vi "Camera  IMAQdx Tester.vi"() -> ()   [LabVIEW 2017]
uses:
  Camera_IMAQdx_class/typedefs/Configuration--Cluster.ctl
  Camera_IMAQdx_class/Camera_IMAQdx.lvclass
  <userlib>/_OpenG.lib/comparison/comparison.llb/Boolean Changed__ogtk.vi
panel:
  in  "Refresh List":bool
  in  "Snap":bool
  in  "Start Stop Grab":bool
  in  "Connect to Camera":bool
  in  "Cameras":u16(ring) items=["VMware Virtual USB Video Device "]
  out "Image":T1(plugin-control)
  in  "OK":bool
  out "Frame Number:":u32
  out "Connected":bool
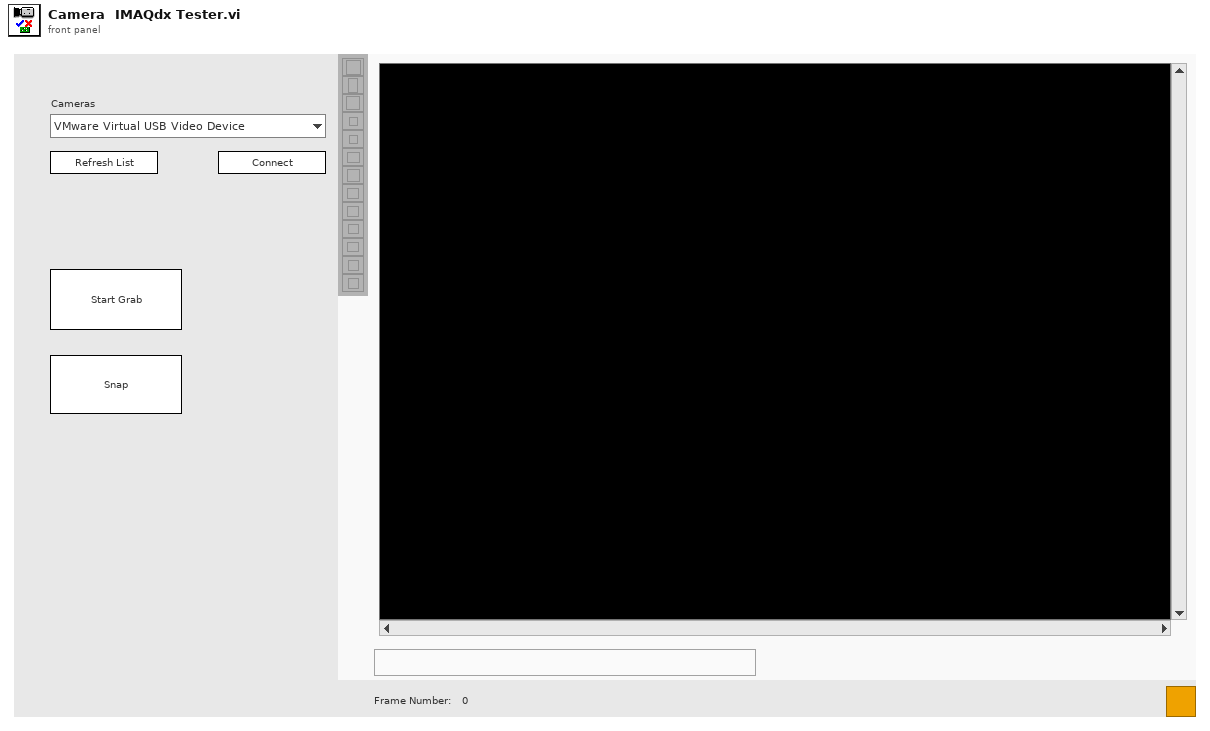
[diagram p1: front panel]
types:
  T1 = typedef "IMAQ Image.ctl" = refnum<image>
  T2 = typedef "Camera_IMAQdx.lvclass/Configuration--Cluster.ctl" = cluster{"Camera Interface Name":string, "Number of Buffers":u32, "Image Name":string, "Image Type":T3}
  T3 = typedef "Image Type" = u32
  T4 = enum32{"invalid app kind", "Development System", "Run Time System", "Student Edition", "Embedded LabVIEW", "Evaluation", "Custom"}
  T5 = enum8{"Enabled", "Disabled", "Disabled and Grayed Out"}
  T6 = enum32{"Invalid", "Standard", "Closed", "Hidden", "Minimized", "Maximized"}
  T7 = cluster{"Core":cluster{"Current VI Reference":refnum<vi>, "Close Panel on Exit?":bool}, "Camera.IMAQdx":refnum<class "Camera_IMAQdx.lvclass">, "All Camera Interfaces":string[], "Connected":bool, "Grabbing":bool}
  T8 = cluster{"Current VI Reference":refnum<vi>, "Close Panel on Exit?":bool}
  T9 = cluster{"Type":u32, "Version":u32, "Flags":u32, "SerialNumberHigh":u32, "SerialNumberLow":u32, "BusType":u32, "InterfaceName":string, "VendorName":string, "ModelName":string, "CameraFileName":string, "CameraAttributeURL":string}[]
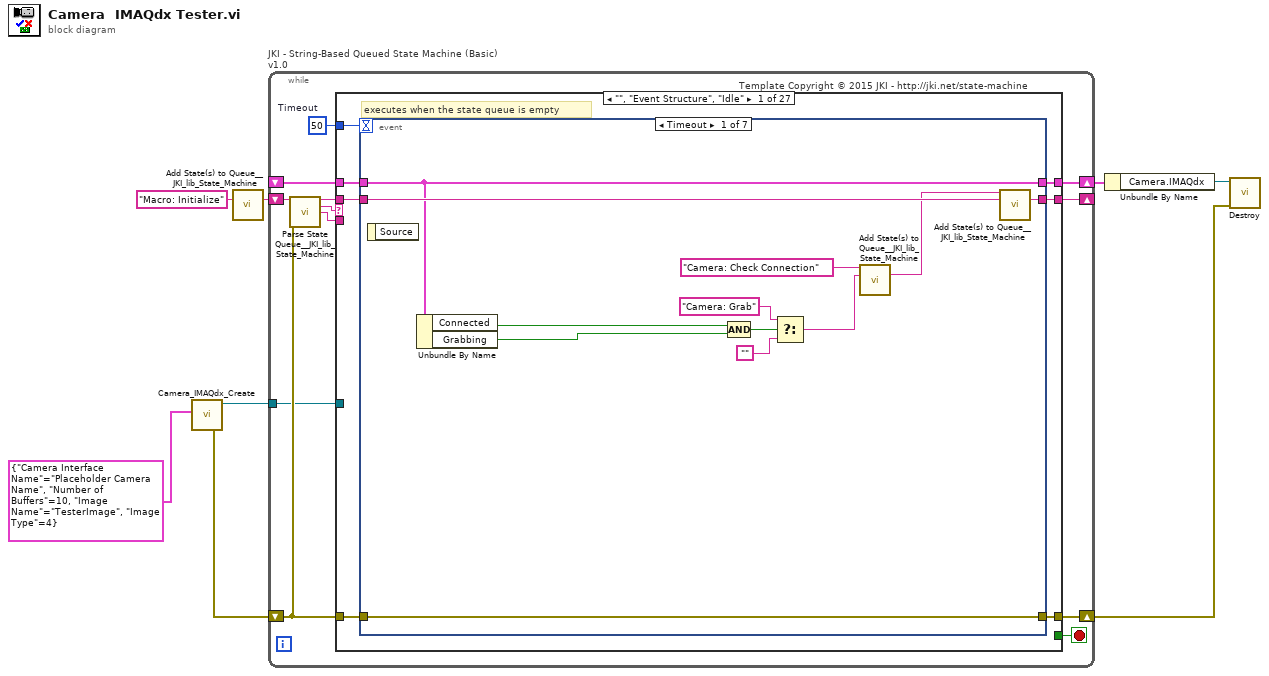
[diagram p0: block diagram]
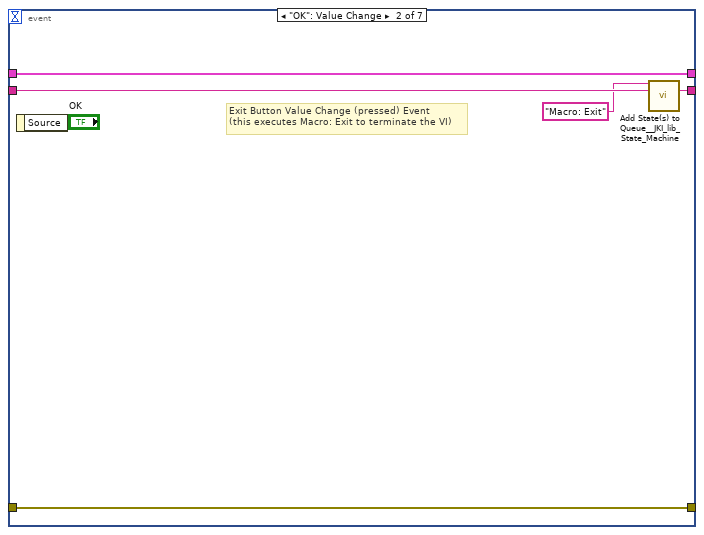
[diagram p2: hidden frame]
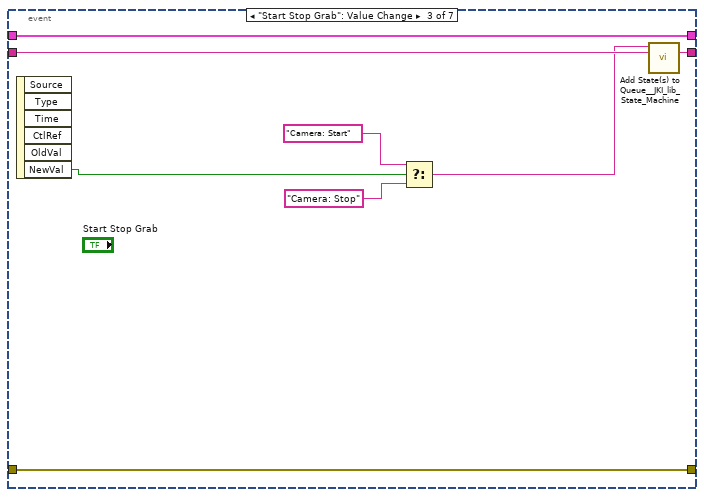
[diagram p3: hidden frame]
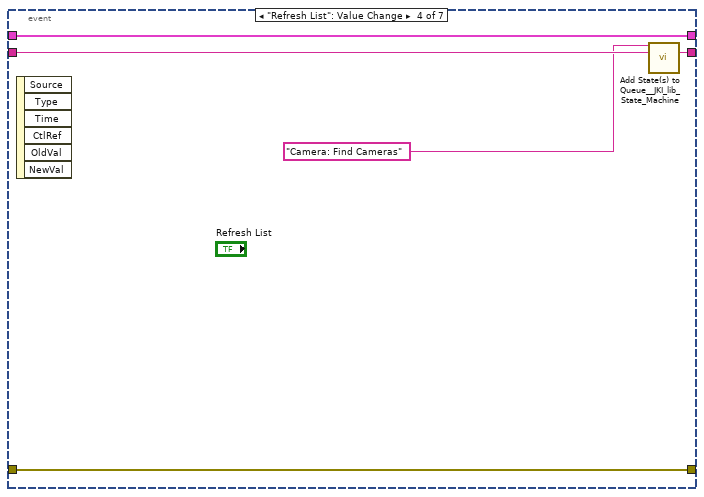
[diagram p4: hidden frame]
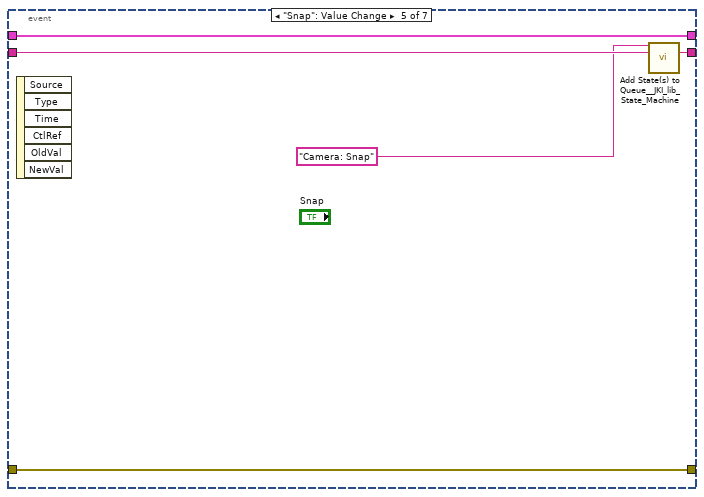
[diagram p5: hidden frame]
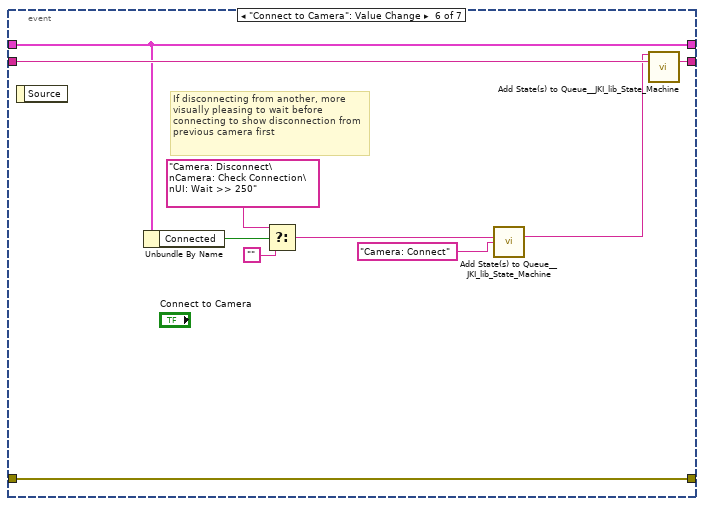
[diagram p6: hidden frame]
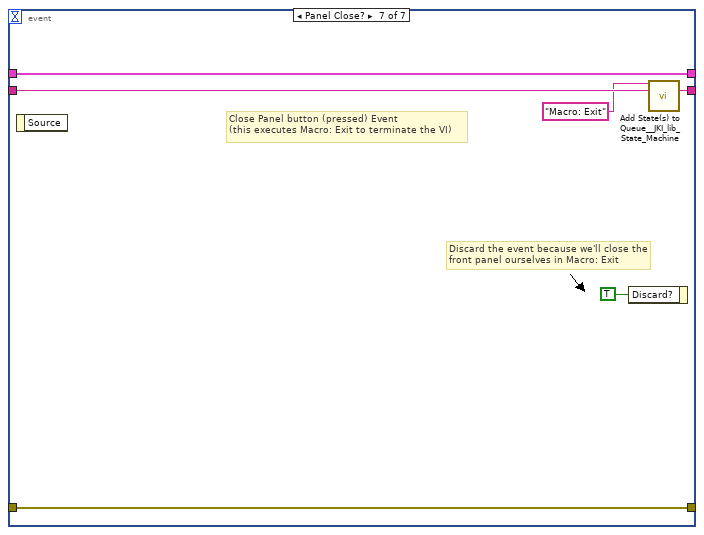
[diagram p7: hidden frame]
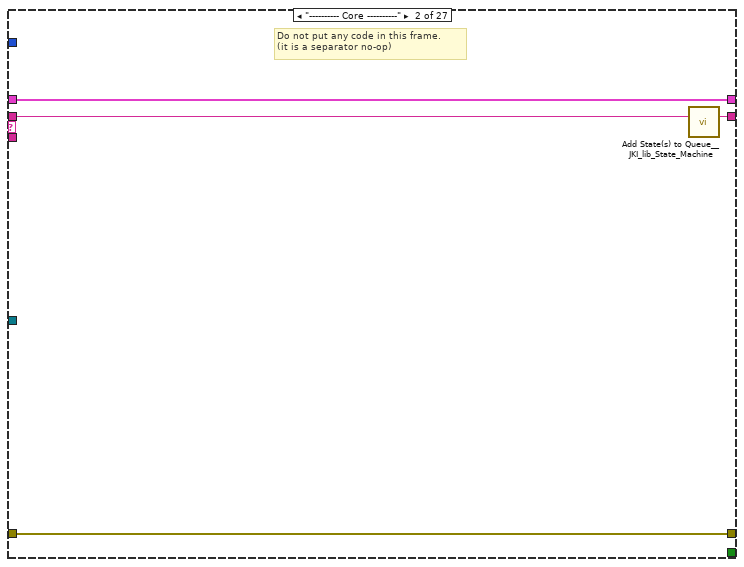
[diagram p8: hidden frame]
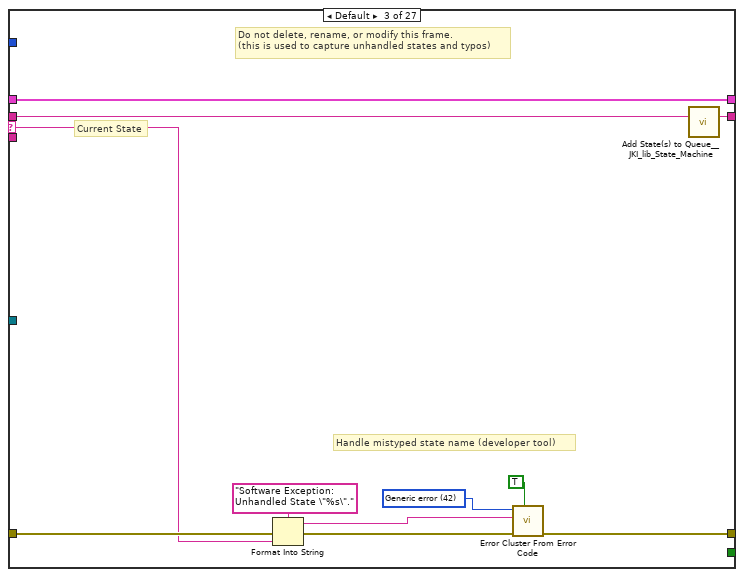
[diagram p9: hidden frame]
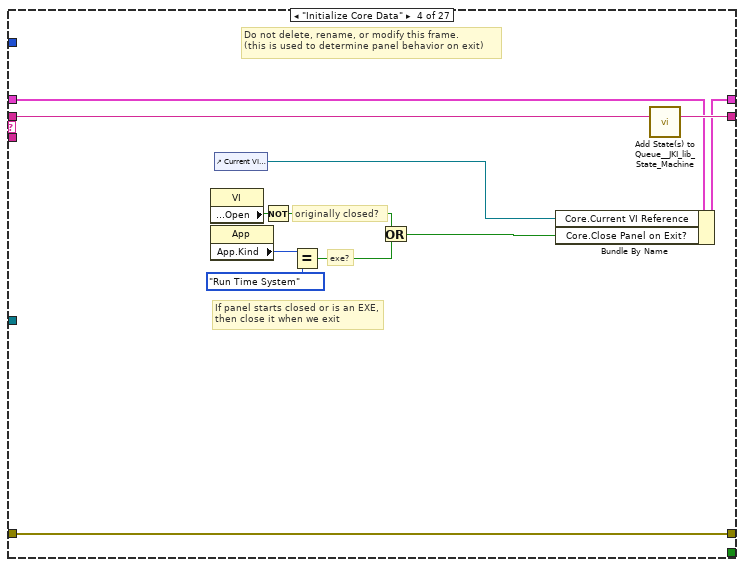
[diagram p10: hidden frame]
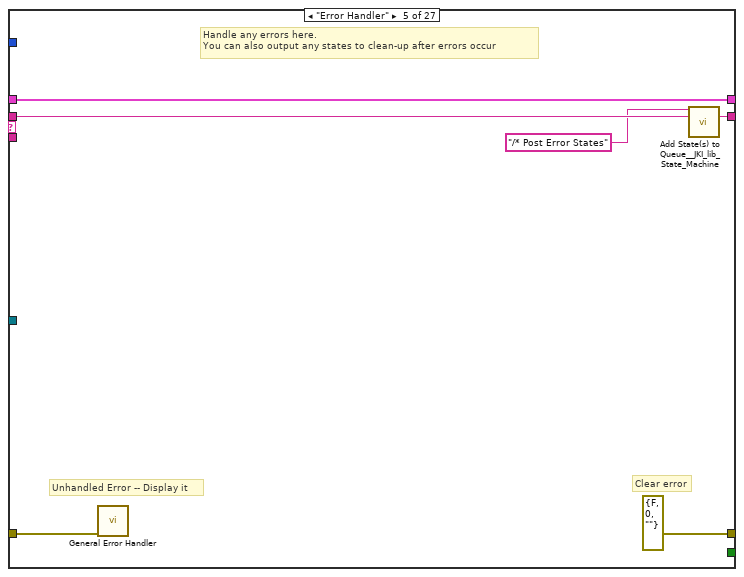
[diagram p11: hidden frame]
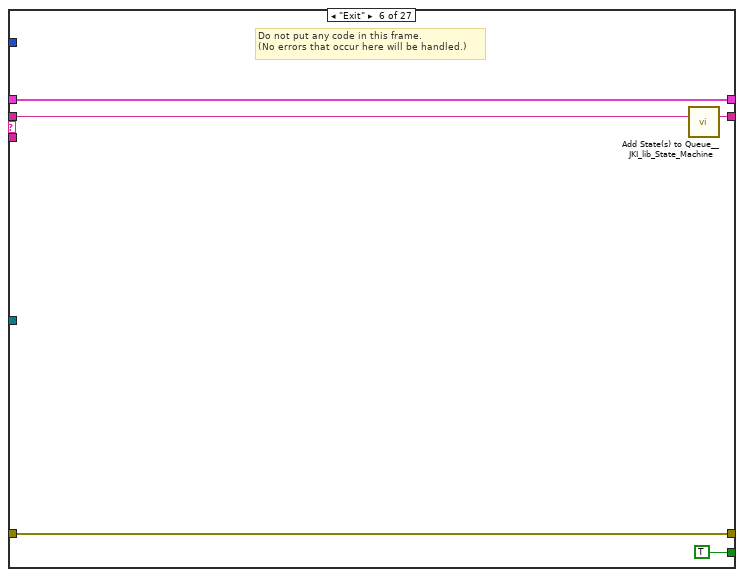
[diagram p12: hidden frame]
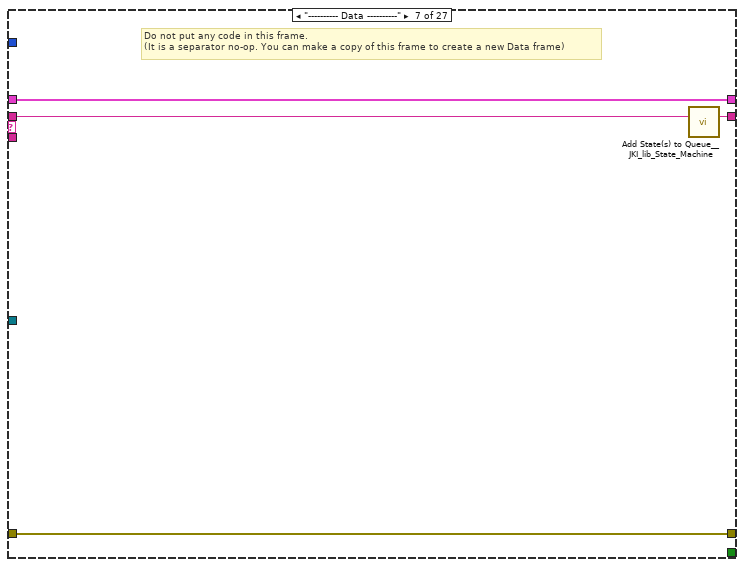
[diagram p13: hidden frame]
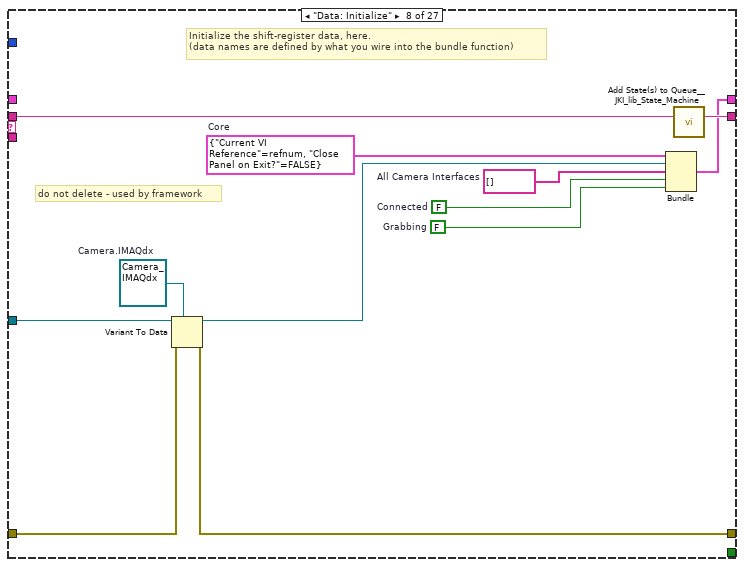
[diagram p14: hidden frame]
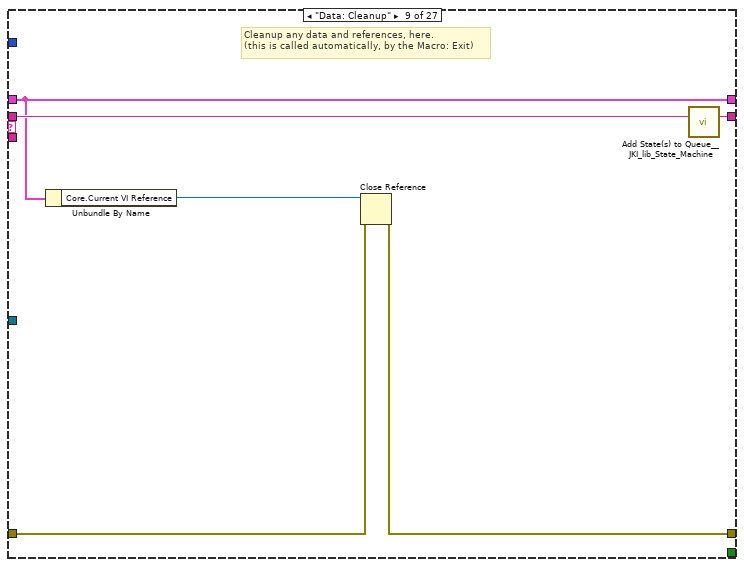
[diagram p15: hidden frame]
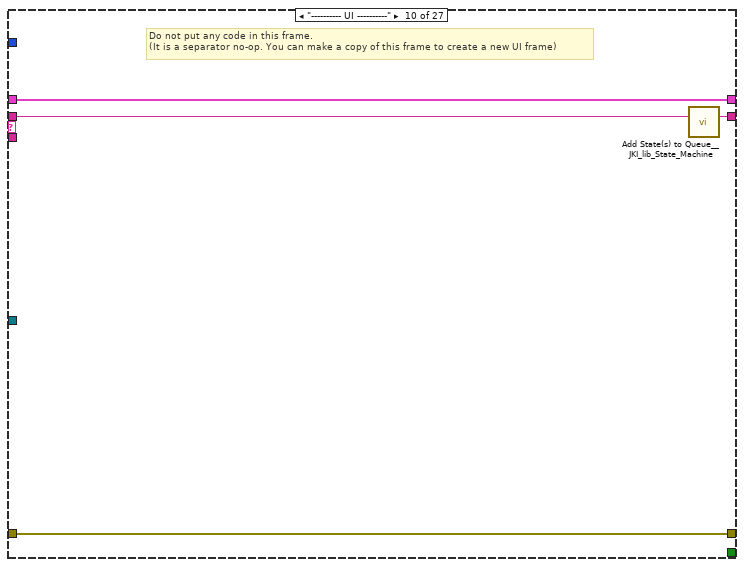
[diagram p16: hidden frame]
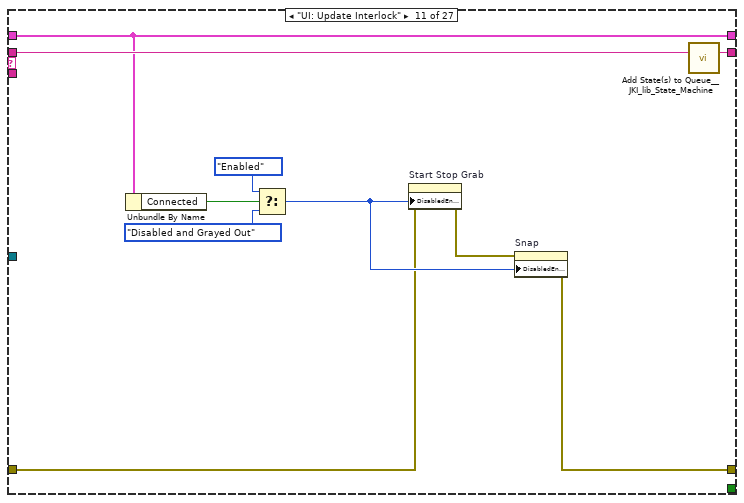
[diagram p17: hidden frame]
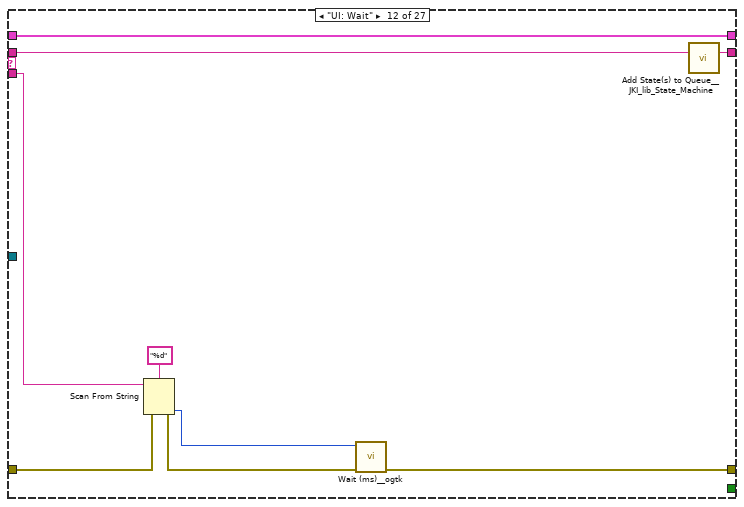
[diagram p18: hidden frame]
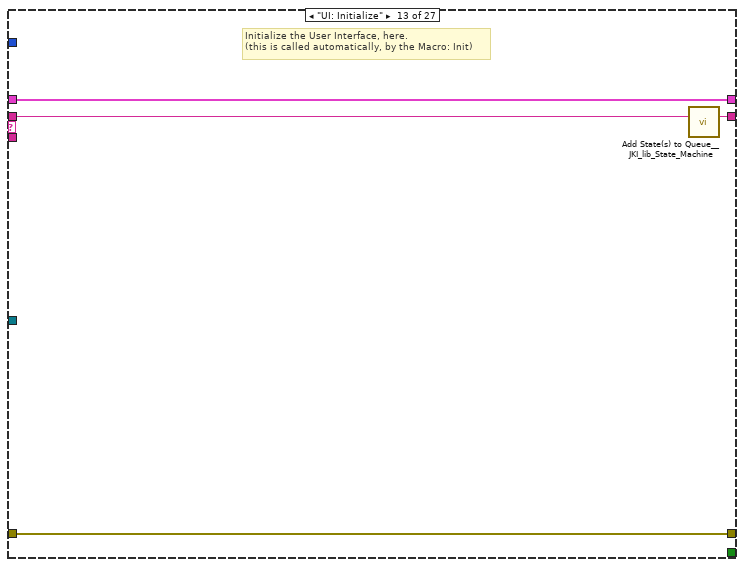
[diagram p19: hidden frame]
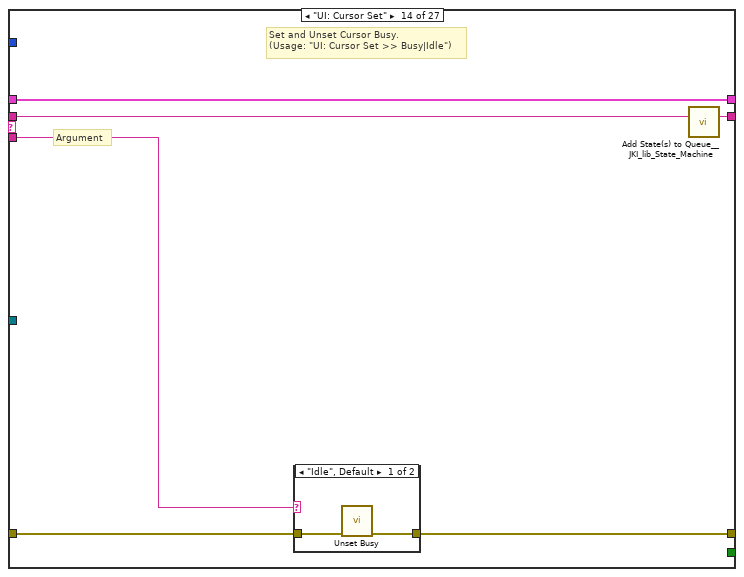
[diagram p20: hidden frame]
diagram:
  n1 = call "Camera_IMAQdx_Create.vi"("Configuration"=T2 {"Camera Interface Name"="Placeholder Camera Name", "Number of Buffers"=10, "Image Name"="TesterImage", "Image Type"=4}) -> ("error out"=w3:errorcluster, "reference out"=w6:refnum<class "Camera_IMAQdx.lvclass">)  [unwired: 9 in]
  n2 = call <vilib>:"Add State(s) to Queue__JKI_lib_State_Machine.vi"("State(s) in (\"\")"="Macro: Initialize") -> ("States Out"=w8:string)  [unwired: 14 in]
  n3 = while "JKI - String-Based Queued State Machine (Basic) v1.0" {
    shift-right: [w13] -> w5
    shift-left: _ -> [w12]
    shift-right: [w16] -> w2
    shift-left: w3 -> [w10]
    shift-right: [w15] -> _
    shift-left: w8 -> [w17]
    tunnel: w6 -> [w9]
    stop <- w14 stop-if-true
    w11 = 50  # Timeout
    # "Template Copyright © 2015 JKI - http://jki.net/state-machine"
    n4 = call <vilib>:"Parse State Queue__JKI_lib_State_Machine.vi"("State Queue"=w17, "Error In (no error)"=w10) -> ("Remaining States"=w19:string, "Current State"=w20:string, "Arguments"=w18:string)  [unwired: 11 in]
    n5 = case shown="\"\", \"Event Structure\", \"Idle\"" w20 {
      selector: w20 -> [_ _ w83 _ _ _ _ _ _ _ _ _ _ _ _ _ _ _ _ _ _ _ _ _ _ _ _]
      tunnel: w19 -> [w27 w82 w87 w105 w111 w116 w120 w132 w138 w142 w152 w161 w165 w171 w182 w208 w213 w232 w236 w244 w251 w263 w272 w281 w292 w309 w315]
      tunnel: w18 -> [_ _ _ _ _ _ _ _ _ _ _ w157 _ w166 w176 _ _ _ _ _ _ _ _ _ _ _ _]
      tunnel: w12 -> [w25 w79 w85 w96 w108 w114 w117 _ w133 w139 w150 w159 w163 w169 w178 w205 w210 w229 w233 w242 w249 w258 w265 w276 w284 w307 w313]
      tunnel: [w24 w80 w89 w102 errorcluster {"status"=FALSE, "code"=0, "source"=""} ("error out") w113 w118 w123 w134 w140 w143 w158 w162 w167 w179 w206 w211 w230 w234 w239 w246 w259 w268 w277 w287 w299 w310] -> w16
      tunnel: w10 -> [w23 w80 w88 w102 w107 w113 w118 w124 w135 w140 w144 w154 w162 w168 w180 w206 w211 w230 w234 w240 w247 w260 w269 w278 w286 w301 w311]
      tunnel: [w26 w81 w86 w104 w110 w115 w119 w131 w137 w141 w151 w160 w164 w170 w181 w207 w212 w231 w235 w243 w250 w262 w271 w280 w291 w308 w314] -> w15
      tunnel: [_ _ _ _ _ TRUE _ _ _ _ _ _ _ _ _ _ _ _ _ _ _ _ _ _ _ _ _] -> w14
      tunnel: [w22 w79 w85 w103 w108 w114 w117 w130 w133 w139 w150 w159 w163 w169 w178 w205 w210 w229 w233 w242 w249 w257 w264 w275 w283 w307 w313] -> w13
      tunnel: w11 -> [w21 _ _ _ _ _ _ _ _ _ _ _ _ _ _ _ _ _ _ _ _ _ _ _ _ _ _]
      tunnel: w9 -> [_ _ _ _ _ _ _ w128 _ _ _ _ _ _ _ _ _ _ _ _ _ _ _ _ _ _ _]
      frame "", "Event Structure", "Idle" {
        # "executes when the state queue is empty"
        n6 = event shown="[0] Timeout" {
          selector: _ -> [_ _ _ _ _ _ _]
          dyn-events: _ -> [_ _ _ _ _ _ _]
          timeout: w21 -> [_ _ _ _ _ _ _]
          tunnel: w27 -> [w39 w44 w52 w57 w62 w72 w78]
          tunnel: [w38 w43 w51 w56 w61 w71 w77] -> w26
          tunnel: w25 -> [w36 w41 w49 w54 w59 w69 w75]
          tunnel: [w37 w42 w50 w55 w60 w70 w76] -> w24
          tunnel: w23 -> [w37 w42 w50 w55 w60 w70 w76]
          tunnel: [w36 w41 w49 w54 w59 w69 w75] -> w22
          event Timeout {
            n7 = event-data() -> ()  [unwired: 1 in, 1 out]
            n8 = Unbundle By Name(w36) -> ("Connected"=w35:bool, "Grabbing"=w34:bool)
            n9 = Compound Arithmetic op=AND(w35, w34) -> (w33:bool)
            n10 = Select(t="Camera: Grab", s=w33, f="") -> (s? t:f=w28:string)
            n11 = call <vilib>:"Add State(s) to Queue__JKI_lib_State_Machine.vi"("State(s) in Front (\"\")"="Camera: Check Connection", "State(s) in (\"\")"=w28) -> ("States Out"=w29:string)  [unwired: 13 in]
            n12 = call <vilib>:"Add State(s) to Queue__JKI_lib_State_Machine.vi"("State(s) in Front (\"\")"=w29, "State(s) in (\"\")"=w39) -> ("States Out"=w38:string)  [unwired: 13 in]
          }
          event "OK": Value Change {
            # "Exit Button Value Change (pressed) Event\n(this executes Macro: Exit to terminate the VI)"
            n13 = event-data() -> ()  [unwired: 1 in, 1 out]
            n14 = call <vilib>:"Add State(s) to Queue__JKI_lib_State_Machine.vi"("State(s) in Front (\"\")"="Macro: Exit", "State(s) in (\"\")"=w44) -> ("States Out"=w43:string)  [unwired: 13 in]
          }
          event "Start Stop Grab": Value Change {
            n15 = event-data() -> ("NewVal"=w46:bool)  [unwired: 1 in, 5 out]
            n16 = Select(t="Camera: Start", s=w46, f="Camera: Stop") -> (s? t:f=w45:string)
            n17 = call <vilib>:"Add State(s) to Queue__JKI_lib_State_Machine.vi"("State(s) in Front (\"\")"=w45, "State(s) in (\"\")"=w52) -> ("States Out"=w51:string)  [unwired: 13 in]
          }
          event "Refresh List": Value Change {
            n18 = event-data() -> ()  [unwired: 1 in, 6 out]
            n19 = call <vilib>:"Add State(s) to Queue__JKI_lib_State_Machine.vi"("State(s) in Front (\"\")"="Camera: Find Cameras", "State(s) in (\"\")"=w57) -> ("States Out"=w56:string)  [unwired: 13 in]
          }
          event "Snap": Value Change {
            n20 = event-data() -> ()  [unwired: 1 in, 6 out]
            n21 = call <vilib>:"Add State(s) to Queue__JKI_lib_State_Machine.vi"("State(s) in Front (\"\")"="Camera: Snap", "State(s) in (\"\")"=w62) -> ("States Out"=w61:string)  [unwired: 13 in]
          }
          event "Connect to Camera": Value Change {
            # "If disconnecting from another, more visually pleasing to wait before connecting to show disconnection from previous camera first"
            n22 = event-data() -> ()  [unwired: 1 in, 1 out]
            n23 = Unbundle By Name(w69) -> ("Connected"=w68:bool)
            n24 = Select(t="Camera: Disconnect\nCamera: Check Connection\nUI: Wait >> 250", s=w68, f="") -> (s? t:f=w65:string)
            n25 = call <vilib>:"Add State(s) to Queue__JKI_lib_State_Machine.vi"("State(s) in (\"\")"=w65, "State(s) at Back (\"\")"="Camera: Connect") -> ("States Out"=w63:string)  [unwired: 13 in]
            n26 = call <vilib>:"Add State(s) to Queue__JKI_lib_State_Machine.vi"("State(s) in Front (\"\")"=w63, "State(s) in (\"\")"=w72) -> ("States Out"=w71:string)  [unwired: 13 in]
          }
          event Panel Close? {
            # "Discard the event because we'll close the front panel ourselves in Macro: Exit"
            # "Close Panel button (pressed) Event\n(this executes Macro: Exit to terminate the VI)"
            n27 = event-data() -> ()  [unwired: 1 in, 1 out]
            n28 = event-data("Discard?"=TRUE) -> ()  [unwired: 1 in, 1 out]
            n29 = call <vilib>:"Add State(s) to Queue__JKI_lib_State_Machine.vi"("State(s) in Front (\"\")"="Macro: Exit", "State(s) in (\"\")"=w78) -> ("States Out"=w77:string)  [unwired: 13 in]
          }
        }
      }
      frame "---------- Core ----------" {
        # "Do not put any code in this frame.\n(it is a separator no-op)"
        n30 = call <vilib>:"Add State(s) to Queue__JKI_lib_State_Machine.vi"("State(s) in (\"\")"=w82) -> ("States Out"=w81:string)  [unwired: 14 in]
      }
      frame Default {
        w92 = 42 items=["No error", "Argument error", "Memory is full", "Out of zone", "End of file", "File already open", "Generic file I/O error", "File not found", "File permission error", "Disk is full", "Duplicate path", "Too many files open", "System feature not enabled", "Resource file not found", "Cannot add resource", "Resource not found", "Image not found", "Image memory error", "Pen does not exist", "Config type invalid", "Config token not found", "Config parse error", "Config memory error", "Bad external code format", "Bad external code offset", "External code not present", "Null window", "Destroy window error", "Null menu", "Print aborted", "Bad print record", "Print driver error", "Windows error during printing", "Memory error during printing", "Print dialog error", "Generic print error", "Invalid device refnum", "Device not found", "Device parameter error", "Device unit error", "Cannot open device", "Device call aborted", "Generic error", "Cancelled by user", "Object ID too low", "Object ID too high", "Object not in heap", "Unknown heap", "Unknown object (invalid DefProc)", "Unknown object (DefProc not in table)", "Message out of range", "Invalid (null) method", "Unknown message", "Manager call not supported", "Bad address", "Network operation in progress", "Network operation timed out", "Connection is busy", "Network attribute not supported", "Network error", "Address in use", "System out of memory", "Connection aborted", "Connection refused", "Not connected", "Already connected", "Connection closed", "Initialization error (interapplication manager)", "Bad occurrence", "Wait on unbound occurrence handler", "Occurrence queue overflow", "Datalog type conflict", "Unused", "Unrecognized type (interapplication manager)", "Memory corrupt", "Failed to make temporary DLL", "Old CIN version", "Drag socket not found", "Failed to load drop-object", "Failed to register OLE object", "Failed to release OLE object", "Format specifier type mismatch", "Unknown format specifier", "Too few format specifiers", "Too many format specifiers", "Scan failed", "Newer CIN version", "Error converting to variant", "Runtime menu error", "Password tampered", "Variant attribute not found", "Incompatible variant data type", "Event data is not available", "Event Store is not present", "Occurrence is not found", "Event Queue is not created", "Event info is not available", "Refnum passed is NULL", "Error retrieving Class GUID", "Error retrieving CoClass GUID", "Error retrieving TypeLib GUID.", "Bad built application magic bytes.", "Specific driver is different from the specific driver associated with the Logical Name.", "There is no session opened to the class driver.", "Max Error", "MAX - Error with config objects", "MAX - Error loading configuration", "MAX - Group not supported"]
        # "Current State"
        # "Do not delete, rename, or modify this frame.\n(this is used to capture unhandled states and typos)"
        # "Handle mistyped state name (developer tool)"
        n31 = Format Into String(format string="Software Exception: Unhandled State \"%s\"." ("message"), error in=w88, w83) -> (resulting string=w91:string, error out=w90:errorcluster)  [unwired: 1 in]
        n32 = call <vilib>:"Error Cluster From Error Code.vi"("show call chain? (False)"=TRUE, "error in (no error)"=w90, "error message (\"\")"=w91, "error code (0)"=w92) -> ("error out"=w89:errorcluster)  [unwired: 5 in]
        n33 = call <vilib>:"Add State(s) to Queue__JKI_lib_State_Machine.vi"("State(s) in (\"\")"=w87) -> ("States Out"=w86:string)  [unwired: 14 in]
      }
      frame "Initialize Core Data" {
        # "Do not delete, rename, or modify this frame.\n(this is used to determine panel behavior on exit)"
        # "originally closed?"
        # "exe?"
        # "If panel starts closed or is an EXE, then close it when we exit"
        n34 = property class="VI"() -> ("Front Panel.Open"=w101:bool)  [unwired: 2 in, 2 out]
        n35 = property class="App"() -> ("App.Kind"=w100:T4)  [unwired: 2 in, 2 out]
        n36 = control-ref of="Current VI Reference"() -> (w94:refnum<vi>)
        n37 = Not(x=w101) -> (.not. x?=w98:bool)
        n38 = Equal?(x=w100, y=T4."Run Time System" ("Application:Kind")) -> (x = y?=w97:bool)
        n39 = Or(x=w98, y=w97) -> (x .or. y?=w95:bool)
        n40 = Bundle By Name(cluster=w96, "Core.Current VI Reference"=w94, "Core.Close Panel on Exit?"=w95) -> (w103:T7)
        n41 = call <vilib>:"Add State(s) to Queue__JKI_lib_State_Machine.vi"("State(s) in (\"\")"=w105) -> ("States Out"=w104:string)  [unwired: 14 in]
      }
      frame "Error Handler" {
        # "Unhandled Error -- Display it"
        # "Handle any errors here.\nYou can also output any states to clean-up after errors occur"
        # "Clear error"
        n42 = call <vilib>:"General Error Handler.vi"("error in (no error)"=w107) -> ()  [unwired: 10 in, 5 out]
        n43 = call <vilib>:"Add State(s) to Queue__JKI_lib_State_Machine.vi"("State(s) in Front (\"\")"="/* Post Error States", "State(s) in (\"\")"=w111) -> ("States Out"=w110:string)  [unwired: 13 in]
      }
      frame "Exit" {
        # "Do not put any code in this frame.\n(No errors that occur here will be handled.)"
        n44 = call <vilib>:"Add State(s) to Queue__JKI_lib_State_Machine.vi"("State(s) in (\"\")"=w116) -> ("States Out"=w115:string)  [unwired: 14 in]
      }
      frame "---------- Data ----------" {
        # "Do not put any code in this frame.\n(It is a separator no-op. You can make a copy of this frame to create a new Data frame)"
        n45 = call <vilib>:"Add State(s) to Queue__JKI_lib_State_Machine.vi"("State(s) in (\"\")"=w120) -> ("States Out"=w119:string)  [unwired: 14 in]
      }
      frame "Data: Initialize" {
        w121 = FALSE  # Grabbing
        w122 = FALSE  # Connected
        w126 = refnum<class "Camera_IMAQdx.lvclass"> refnum  # Camera.IMAQdx
        w127 = string[] []  # All Camera Interfaces
        w129 = T8 {"Current VI Reference"=refnum, "Close Panel on Exit?"=FALSE}  # Core
        # "do not delete - used by framework"
        # "Initialize the shift-register data, here.\n(data names are defined by what you wire into the bundle function)"
        n46 = Variant To Data(error in=w124, type=w126, Variant=w128) -> (data=w125:refnum<class "Camera_IMAQdx.lvclass">, error out=w123:errorcluster)
        n47 = Bundle("Core"=w129, "Camera.IMAQdx"=w125, "All Camera Interfaces"=w127, "Connected"=w122, "Grabbing"=w121) -> (w130:T7)  [unwired: 1 in]
        n48 = call <vilib>:"Add State(s) to Queue__JKI_lib_State_Machine.vi"("State(s) in (\"\")"=w132) -> ("States Out"=w131:string)  [unwired: 14 in]
      }
      frame "Data: Cleanup" {
        # "Cleanup any data and references, here.\n(this is called automatically, by the Macro: Exit)"
        n49 = Unbundle By Name(w133) -> ("Core.Current VI Reference"=w136:refnum<vi>)
        n50 = Close Reference(reference=w136, error in (no error)=w135) -> (error out=w134:errorcluster)
        n51 = call <vilib>:"Add State(s) to Queue__JKI_lib_State_Machine.vi"("State(s) in (\"\")"=w138) -> ("States Out"=w137:string)  [unwired: 14 in]
      }
      frame "---------- UI ----------" {
        # "Do not put any code in this frame.\n(It is a separator no-op. You can make a copy of this frame to create a new UI frame)"
        n52 = call <vilib>:"Add State(s) to Queue__JKI_lib_State_Machine.vi"("State(s) in (\"\")"=w142) -> ("States Out"=w141:string)  [unwired: 14 in]
      }
      frame "UI: Update Interlock" {
        n53 = Unbundle By Name(w150) -> ("Connected"=w149:bool)
        n54 = Select(t=T5."Enabled" ("Disabled"), s=w149, f=T5."Disabled and Grayed Out" ("Disabled")) -> (s? t:f=w146:T5)
        n55 = property on="Start Stop Grab" class="Bool (strict)"(error in=w144, "DisabledEnum"=w146) -> (error out=w145:errorcluster)  [unwired: 1 in, 1 out]
        n56 = property on="Snap" class="Bool"(error in=w145, "DisabledEnum"=w146) -> (error out=w143:errorcluster)  [unwired: 1 in, 1 out]
        n57 = call <vilib>:"Add State(s) to Queue__JKI_lib_State_Machine.vi"("State(s) in (\"\")"=w152) -> ("States Out"=w151:string)  [unwired: 14 in]
      }
      frame "UI: Wait" {
        n58 = Scan From String(format string="%d", input string=w157, error in=w154) -> (error out=w153:errorcluster, output 1=w155:i32)  [unwired: 2 in, 2 out]
        n59 = call <userlib>:"Wait (ms)__ogtk.vi"("error in (no error)"=w153, "milliseconds to wait"=w155) -> ("error out"=w158:errorcluster)  [unwired: 8 in, 1 out]
        n60 = call <vilib>:"Add State(s) to Queue__JKI_lib_State_Machine.vi"("State(s) in (\"\")"=w161) -> ("States Out"=w160:string)  [unwired: 14 in]
      }
      frame "UI: Initialize" {
        # "Initialize the User Interface, here.\n(this is called automatically, by the Macro: Init)"
        n61 = call <vilib>:"Add State(s) to Queue__JKI_lib_State_Machine.vi"("State(s) in (\"\")"=w165) -> ("States Out"=w164:string)  [unwired: 14 in]
      }
      frame "UI: Cursor Set" {
        # "Argument"
        # "Set and Unset Cursor Busy.\n(Usage: \"UI: Cursor Set >> Busy|Idle\")"
        n62 = case shown="\"Idle\", Default" w166 {
          tunnel: w168 -> [w173 w175]
          tunnel: [w172 w174] -> w167
          frame "Idle", Default {
            n63 = call <vilib>:"Unset Busy.vi"("error in (no error)"=w173) -> ("error out"=w172:errorcluster)  [unwired: 10 in]
          }
          frame "Busy" {
            n64 = call <vilib>:"Set Busy.vi"("error in (no error)"=w175) -> ("error out"=w174:errorcluster)  [unwired: 9 in, 1 out]
          }
        }
        n65 = call <vilib>:"Add State(s) to Queue__JKI_lib_State_Machine.vi"("State(s) in (\"\")"=w171) -> ("States Out"=w170:string)  [unwired: 14 in]
      }
      frame "UI: Front Panel State" {
        # "Argument"
        # "Set Front Panel Open or Closed\n(Usage: \"UI: Front Panel State >> Open|Close\")"
        n66 = Unbundle By Name(w178) -> ("Core.Current VI Reference"=w177:refnum<vi>)
        n67 = case shown="\"Open\", Default" w176 {
          tunnel: w180 -> [w186 w199]
          tunnel: [w188 w200] -> w179
          tunnel: w177 -> [w187 w197]
          frame "Open", Default {
            n68 = property class="VI"(reference=w187, error in=w186) -> (reference out=w184:refnum<vi>, error out=w185:errorcluster, "Front Panel.Open"=w183:bool)
            n69 = case shown="False" w183 {
              tunnel: [w191 w194] -> w188
              tunnel: w185 -> [w190 w194]
              tunnel: w184 -> [w189 _]
              frame False {
                n70 = invoke class="VI" method="FP.Open"(reference=w189, error in=w190, "Activate"=TRUE, "State"=T6."Standard") -> (error out=w191:errorcluster)  [unwired: 1 in, 4 out]
              }
              frame True {
              }
            }
          }
          frame "Close" {
            n71 = property class="VI"(reference=w197, error in=w199) -> (reference out=w196:refnum<vi>, error out=w198:errorcluster, "Front Panel.Open"=w195:bool)
            n72 = case shown="True" w195 {
              tunnel: [w201 w204] -> w200
              tunnel: w198 -> [w201 w203]
              tunnel: w196 -> [_ w202]
              frame False {
              }
              frame True {
                n73 = invoke class="VI" method="FP.Close"(reference=w202, error in=w203) -> (error out=w204:errorcluster)  [unwired: 1 in, 2 out]
              }
            }
          }
        }
        n74 = call <vilib>:"Add State(s) to Queue__JKI_lib_State_Machine.vi"("State(s) in (\"\")"=w182) -> ("States Out"=w181:string)  [unwired: 14 in]
      }
      frame "---------- Macro ----------" {
        # "Do not put any code in this frame.\n(It is a separator no-op. You can make a copy of this frame to create a new Macro frame)"
        n75 = call <vilib>:"Add State(s) to Queue__JKI_lib_State_Machine.vi"("State(s) in (\"\")"=w208) -> ("States Out"=w207:string)  [unwired: 14 in]
      }
      frame "Macro: Initialize" {
        # "Initialization Macro\n(This is called once, when the VI starts)"
        n76 = call <vilib>:"Add State(s) to Queue__JKI_lib_State_Machine.vi"("State(s) in Front (\"\")"="Data: Initialize\nInitialize Core Data\nUI: Initialize\nCamera: Find Cameras\nUI: Update Interlock\nUI: Front Panel State >> Open", "State(s) in (\"\")"=w213) -> ("States Out"=w212:string)  [unwired: 13 in]
      }
      frame "Macro: Exit" {
        # "Exit Macro\n(This is called once, when the VI exits)"
        n77 = Unbundle By Name(w229) -> ("Grabbing"=w218:bool, "Connected"=w217:bool, "Core.Close Panel on Exit?"=w228:bool)
        n78 = Select(t="Camera: Stop", s=w218, f="") -> (s? t:f=w216:string)
        n79 = Select(t="Camera: Disconnect", s=w217, f="") -> (s? t:f=w215:string)
        n80 = Select(t="UI: Front Panel State >> Close", s=w228, f="") -> (s? t:f=w225:string)
        n81 = call <vilib>:"Add State(s) to Queue__JKI_lib_State_Machine.vi"("State(s) in Front (\"\")"=w216, "State(s) in (\"\")"=w215) -> ("States Out"=w214:string)  [unwired: 13 in]
        n82 = call <vilib>:"Add State(s) to Queue__JKI_lib_State_Machine.vi"("State(s) in Front (\"\")"=w214, "State(s) in (\"\")"=w225, "State(s) at Back (\"\")"="Data: Cleanup\nExit") -> ("States Out"=w223:string)  [unwired: 12 in]
        n83 = call <vilib>:"Add State(s) to Queue__JKI_lib_State_Machine.vi"("State(s) in Front (\"\")"=w223, "State(s) in (\"\")"=w232) -> ("States Out"=w231:string)  [unwired: 13 in]
      }
      frame "---------- Camera ----------" {
        # "Template Separator\n(You can make a copy of, or modify, this frame)"
        n84 = call <vilib>:"Add State(s) to Queue__JKI_lib_State_Machine.vi"("State(s) in (\"\")"=w236) -> ("States Out"=w235:string)  [unwired: 14 in]
      }
      frame "Camera: Grab" {
        n85 = Unbundle By Name(w242) -> ("Camera.IMAQdx"=w241:refnum<class "Camera_IMAQdx.lvclass">)
        n86 = call-dynamic "Grab.vi"("error in (no error)"=w240, "reference in"=w241) -> ("error out"=w239:errorcluster, "Frame Number"=→"Frame Number:":u32, "Image Out"=→"Image":T1)  [unwired: 6 in, 1 out]
        n87 = call <vilib>:"Add State(s) to Queue__JKI_lib_State_Machine.vi"("State(s) in (\"\")"=w244) -> ("States Out"=w243:string)  [unwired: 14 in]
      }
      frame "Camera: Snap" {
        n88 = Unbundle By Name(w249) -> ("Camera.IMAQdx"=w248:refnum<class "Camera_IMAQdx.lvclass">)
        n89 = call-dynamic "Snap.vi"("error in (no error)"=w247, "reference in"=w248) -> ("error out"=w246:errorcluster, "Image Out"=w245:T1)  [unwired: 7 in, 1 out]
        n90 = local write "Image"(w245) -> ()
        n91 = call <vilib>:"Add State(s) to Queue__JKI_lib_State_Machine.vi"("State(s) in (\"\")"=w251) -> ("States Out"=w250:string)  [unwired: 14 in]
      }
      frame "Camera: Check Connection" {
        n92 = Unbundle By Name(w258) -> ("Camera.IMAQdx"=w261:refnum<class "Camera_IMAQdx.lvclass">)
        n93 = call-dynamic "GetConnected.vi"("error in (no error)"=w260, "reference in"=w261) -> ("error out"=w259:errorcluster, "Connected"=w256:bool)  [unwired: 7 in, 1 out]
        "Connected" <- w256
        n94 = call-poly <userlib>:"Data Changed__ogtk.vi"("Boolean"=w256) -> ("Changed"=w255:bool)
        n95 = Bundle By Name(cluster=w258, "Connected"=w256) -> (w257:T7)
        n96 = Select(t="UI: Update Interlock", s=w255, f="") -> (s? t:f=w252:string)
        n97 = call <vilib>:"Add State(s) to Queue__JKI_lib_State_Machine.vi"("State(s) in Front (\"\")"=w252, "State(s) in (\"\")"=w263) -> ("States Out"=w262:string)  [unwired: 13 in]
      }
      frame "Camera: Start" {
        n98 = Unbundle By Name(w265) -> ("Camera.IMAQdx"=w270:refnum<class "Camera_IMAQdx.lvclass">)
        n99 = call-dynamic "StartAcquisition.vi"("error in (no error)"=w269, "reference in"=w270) -> ("error out"=w268:errorcluster)  [unwired: 8 in, 1 out]
        n100 = Unbundle By Name(w268) -> ("status"=w267:bool)
        n101 = Not(x=w267) -> (.not. x?=w266:bool)
        n102 = Bundle By Name(cluster=w265, "Grabbing"=w266) -> (w264:T7)
        n103 = call <vilib>:"Add State(s) to Queue__JKI_lib_State_Machine.vi"("State(s) in (\"\")"=w272) -> ("States Out"=w271:string)  [unwired: 14 in]
      }
      frame "Camera: Stop" {
        n104 = Unbundle By Name(w276) -> ("Camera.IMAQdx"=w279:refnum<class "Camera_IMAQdx.lvclass">)
        n105 = call-dynamic "StopAcquisition.vi"("error in (no error)"=w278, "reference in"=w279) -> ("error out"=w277:errorcluster)  [unwired: 8 in, 1 out]
        n106 = local write "Frame Number:"(u32 0 ("Frame Number:")) -> ()
        n107 = Bundle By Name(cluster=w276, "Grabbing"=FALSE) -> (w275:T7)
        n108 = call <vilib>:"Add State(s) to Queue__JKI_lib_State_Machine.vi"("State(s) in (\"\")"=w281) -> ("States Out"=w280:string)  [unwired: 14 in]
      }
      frame "Camera: Find Cameras" {
        n109 = Unbundle By Name(w284) -> ("Camera.IMAQdx"=w290:refnum<class "Camera_IMAQdx.lvclass">)
        n110 = call "FindCameras.vi"("error in (no error)"=w286, "reference in"=w290) -> ("error out"=w285:errorcluster, "Camera Information Array"=w289:T9)  [unwired: 7 in, 1 out]
        n111 = for {
          tunnel: w289 -> [w298] mode=indexing
          tunnel: [w294] -> w288 mode=indexing
          tunnel: [w293] -> w282 mode=indexing
          n112 = Unbundle By Name(w298) -> ("InterfaceName"=w293:string, "VendorName"=w297:string, "ModelName"=w295:string)
          n113 = call <vilib>:"Space Constant.vi"() -> ("String"=w296:string)
          n114 = Concatenate Strings(w297, w296, w295) -> (w294:string)
        }
        n115 = Bundle By Name(cluster=w284, "All Camera Interfaces"=w282) -> (w283:T7)
        n116 = property on="Cameras" class="Ring (strict)"(error in=w285, "Strings []"=w288) -> (error out=w287:errorcluster)  [unwired: 1 in, 1 out]
        n117 = call <vilib>:"Add State(s) to Queue__JKI_lib_State_Machine.vi"("State(s) in (\"\")"=w292) -> ("States Out"=w291:string)  [unwired: 14 in]
      }
      frame "Camera: Connect" {
        n118 = Unbundle By Name(w307) -> ("Camera.IMAQdx"=w306:refnum<class "Camera_IMAQdx.lvclass">, "All Camera Interfaces"=w304:string[])
        n119 = Index Array(array=w304, index="Cameras") -> (element=w302:string)
        n120 = call "SetCameraInterfaceName.vi"("error in (no error)"=w301, "Camera Interface Name"=w302, "reference in"=w306) -> ("error out"=w300:errorcluster, "reference out"=w305:refnum<class "Camera_IMAQdx.lvclass">)  [unwired: 7 in]
        n121 = call-dynamic "Connect.vi"("error in (no error)"=w300, "reference in"=w305) -> ("error out"=w299:errorcluster)  [unwired: 8 in, 1 out]
        n122 = call <vilib>:"Add State(s) to Queue__JKI_lib_State_Machine.vi"("State(s) in (\"\")"=w309) -> ("States Out"=w308:string)  [unwired: 14 in]
      }
      frame "Camera: Disconnect" {
        n123 = Unbundle By Name(w313) -> ("Camera.IMAQdx"=w312:refnum<class "Camera_IMAQdx.lvclass">)
        n124 = call-dynamic "Disconnect.vi"("error in (no error)"=w311, "reference in"=w312) -> ("error out"=w310:errorcluster)  [unwired: 8 in, 1 out]
        n125 = call <vilib>:"Add State(s) to Queue__JKI_lib_State_Machine.vi"("State(s) in (\"\")"=w315) -> ("States Out"=w314:string)  [unwired: 14 in]
      }
    }
  }
  n126 = Unbundle By Name(w5) -> ("Camera.IMAQdx"=w4:refnum<class "Camera_IMAQdx.lvclass">)
  n127 = call-dynamic "Destroy.vi"("error in (no error)"=w2, "reference in"=w4) -> ()  [unwired: 8 in, 2 out]
